vi "gyro_flag.vi"() -> ()   [LabVIEW 2019]
uses:
  <vilib>/Utility/file.llb/Read Delimited Spreadsheet (string).vi
  <vilib>/Analysis/NI_AALBase.lvlib
  <vilib>/Utility/file.llb/Write Delimited Spreadsheet (string).vi
panel:
  out "XY Graph":cluster{timestamp[], "Y":dbl[]}[](graph)
  in  "reset":bool
  out "voltage over time":waveform(dbl)(graph)
  out "charge [V]":dbl
  in  "invert":bool
  out "all rows":string[][](array[string])
  in  "Race time":string
  in  "Other":string
  in  "Enviroment":string(combo)
  in  "Tiredness":string(combo)
  in  "Technique":string(combo)
  in  "Orient":string(combo)
  in  "Ship type":string(combo)
  in  "End Comment":bool
  in  "Type":string(combo)
  in  "?":bool
  in  "Felvesz":bool
  out "csv path":path
  in  "Flag":string(combo)
  out "Timestamp":timestamp
  in  "path to binary file":path=path "C:/Users/Lenovo/Desktop/szakdoga/data"
  # "RESET"
  # "ZOOM"
  # "CURSOR"
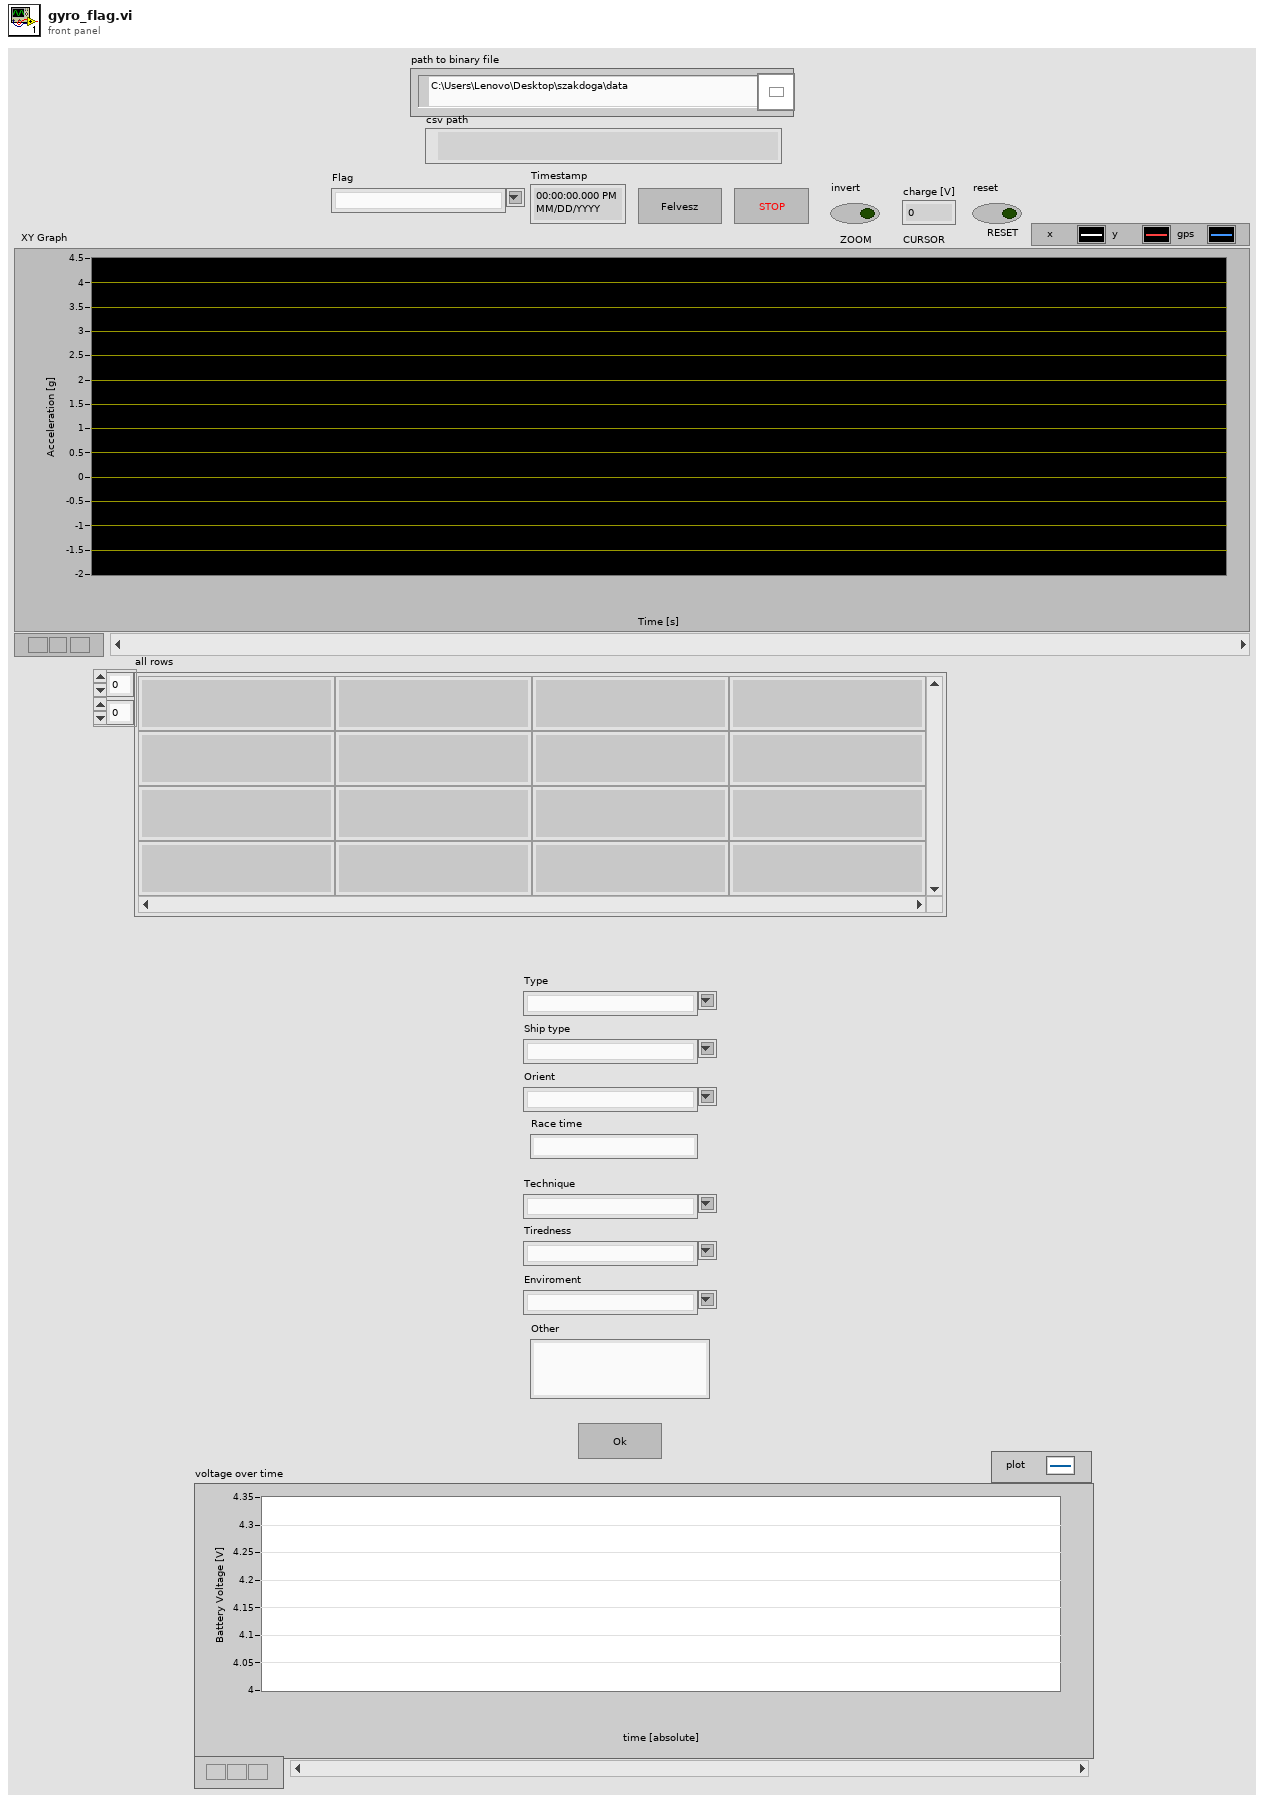
[diagram p1: front panel]
types:
  T1 = enum16{"open", "replace", "create", "open or create", "replace or create", "replace or create with confirmation"}
  T2 = typedef "control_time_informations.ctl" = cluster{"starting time":timestamp, "ending time":timestamp, "dt[s]":dbl, "sampling rate [Hz]":dbl, "length":dbl}
  T3 = typedef "control_all_in_one_package.ctl" = cluster{"memory structure":T4, "actigraph settings":T5, "time informations":T2, "measurement data":T6}
  T4 = typedef "control_memory_structure.ctl" = cluster{"length of metadata [byte]":i32, "length of page [byte]":i32, "length of measurement data on page [byte]":i32, "length of dataset [byte]":i32}
  T5 = typedef "control_measurement_settings.ctl" = cluster{"sampling frequency [Hz]":dbl, "measurement interval [± g]":i32, "high precision?":bool, "number of pages":i32, "rate code":i32, "range code":i32, "id":i32}
  T6 = typedef "control_measurement_data.ctl" = cluster{"number of samples per axis":i32, "timestamp array":dbl[], "offset array":dbl[], "x, y, z axis data":waveform(dbl)[], "normalised magnitude of acceleartion vectors":waveform(dbl), "calibration coefficients":T7, "statistics":T8, "battery voltage":waveform(dbl), "magnitude of acceleartion vectors":waveform(dbl)}
  T7 = typedef "control_calibration_coefficients.ctl" = cluster{"Sx":dbl, "Ox":dbl, "Sy":dbl, "Oy":dbl, "Sz":dbl, "Oz":dbl}
  T8 = typedef "control_statistics.ctl" = cluster{"mean of x axis acceleration":dbl, "standard devation of x axis acceleration":dbl, "mean of y axis acceleration":dbl, "standard devation of y axis acceleration":dbl, "mean of z axis acceleration":dbl, "standard devation of z axis acceleration":dbl, "mean of normalised magnitude of acceleration":dbl, "standard devation of normalised magnitude of acceleration":dbl}
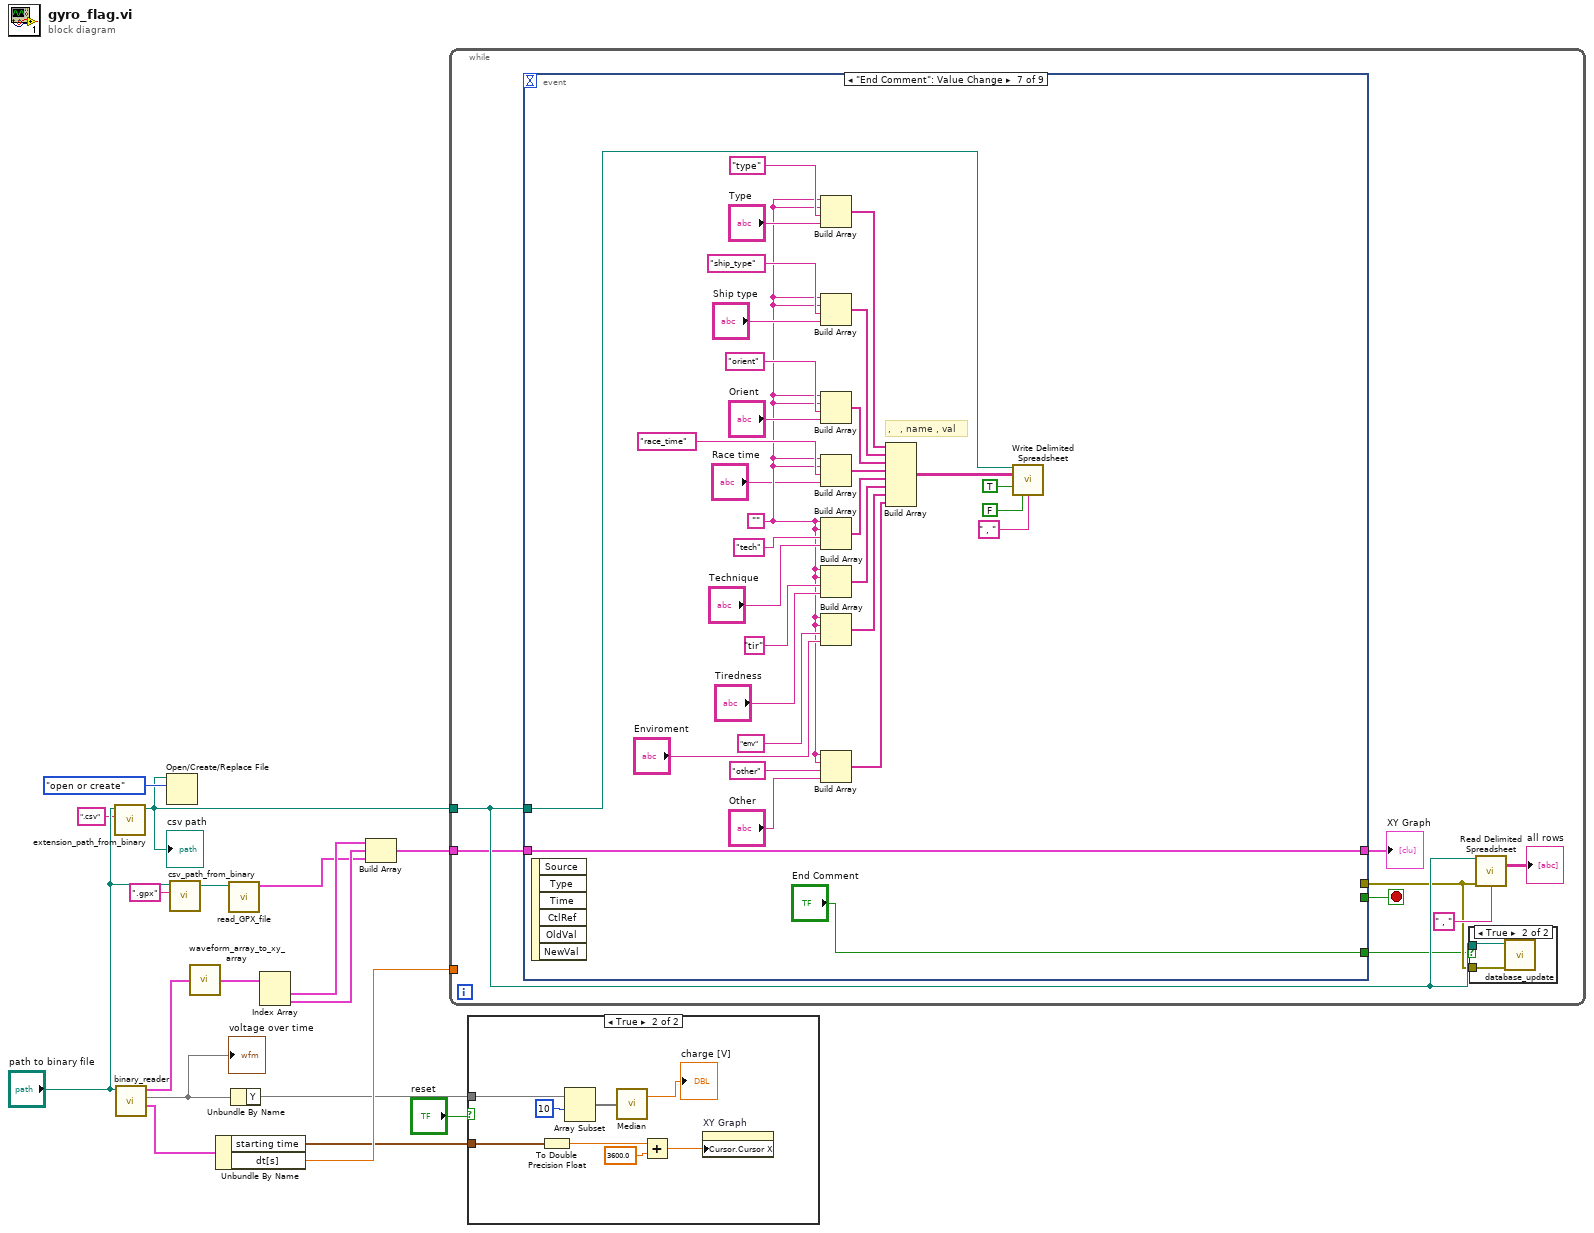
[diagram p0: block diagram]
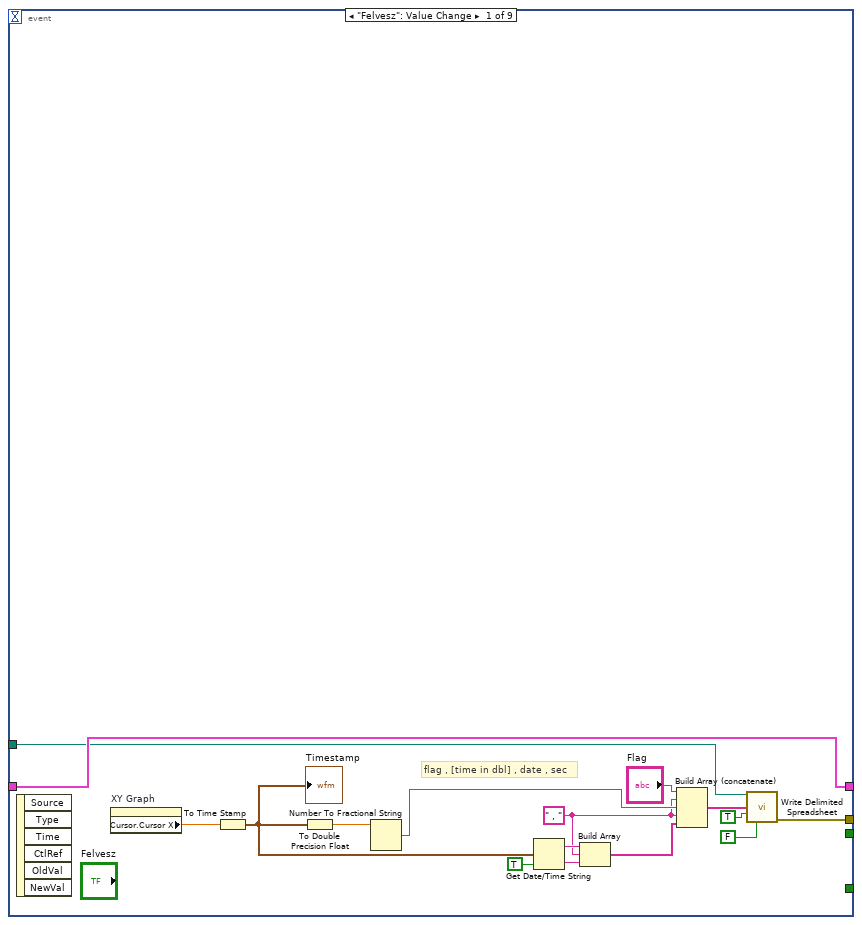
[diagram p4: hidden frame]
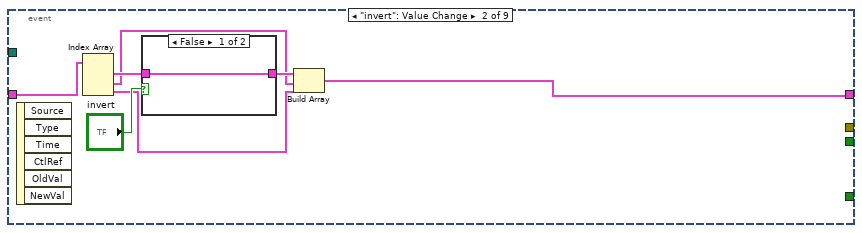
[diagram p5: hidden frame]
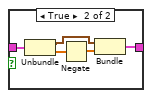
[diagram p6: hidden frame]
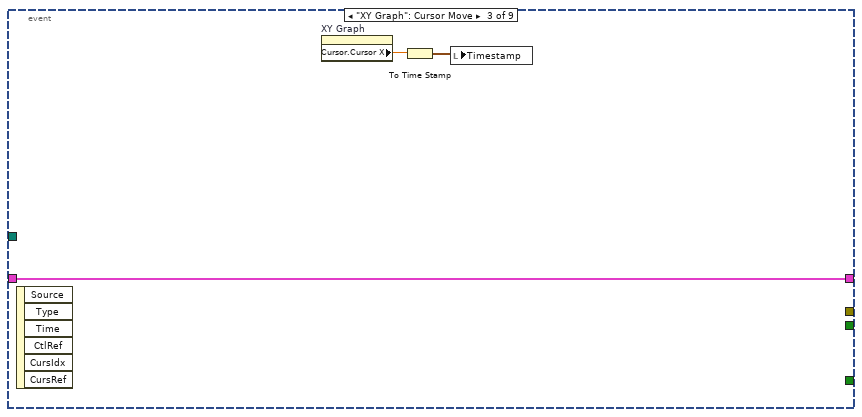
[diagram p7: hidden frame]
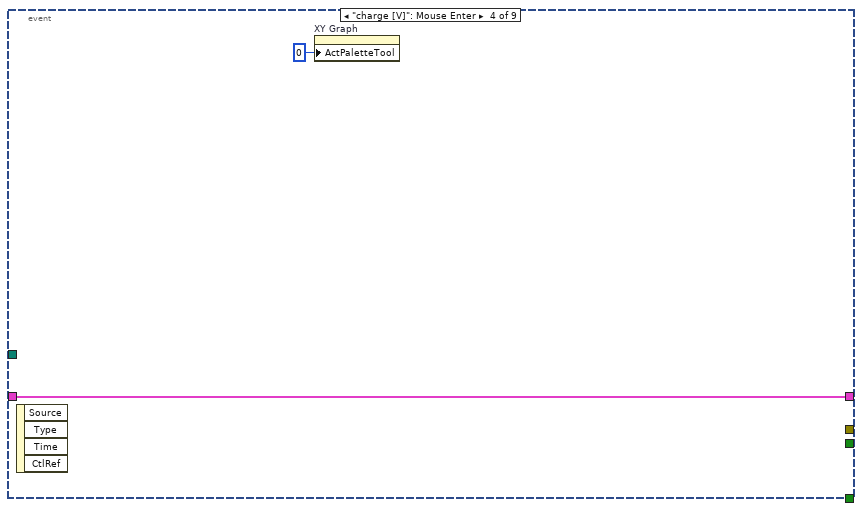
[diagram p8: hidden frame]
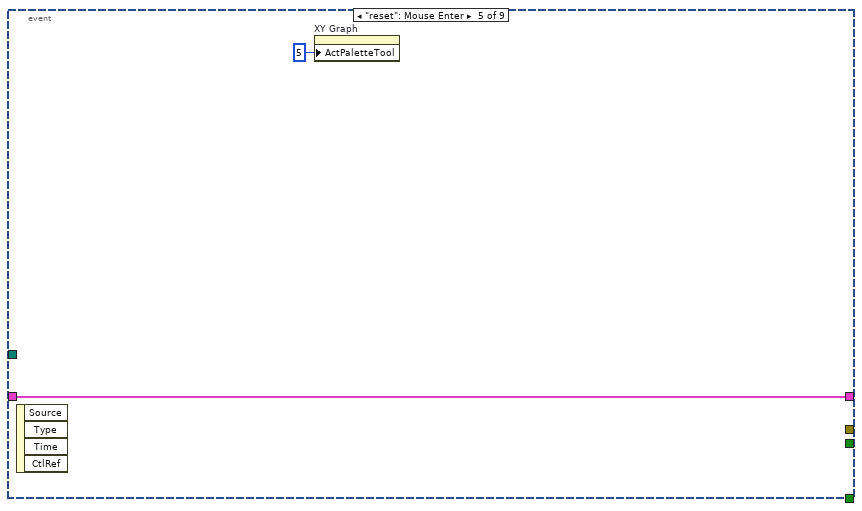
[diagram p9: hidden frame]
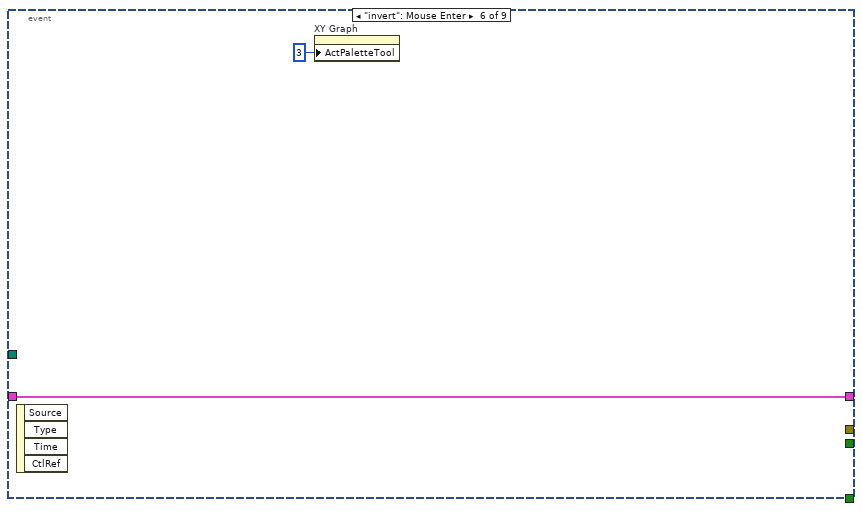
[diagram p10: hidden frame]
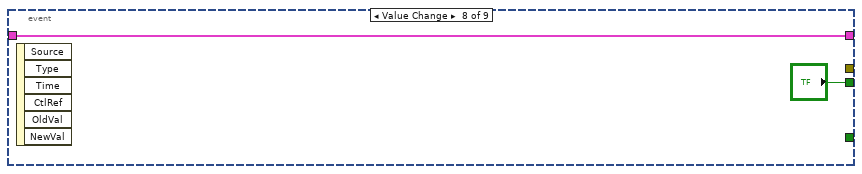
[diagram p11: hidden frame]
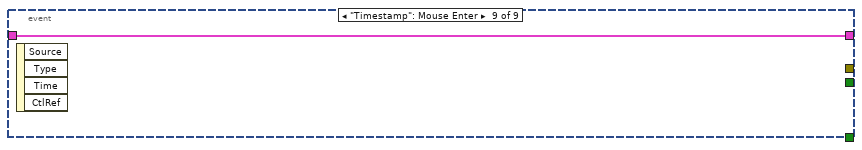
[diagram p12: hidden frame]
diagram:
  n1 = call "extension_path_from_binary.vi"("extension"=".csv", "path to binary file"="path to binary file") -> ("path to csv"=w1:path)  [unwired: 9 in]
  "csv path" <- w1
  n2 = call "binary_reader.vi"("path to binary file"="path to binary file") -> ("time informations"=w12:T2, 2:w11, "all in one package"=w5:T3)  [unwired: 6 in, 1 out]
  "voltage over time" <- w11
  n3 = Open/Create/Replace File(file path (use dialog)=w1, operation (0:open)=T1."open or create") -> ()  [unwired: 4 in, 3 out]
  n4 = call "csv_path_from_binary.vi"("extension"=".gpx", "path to binary file"="path to binary file") -> ("path to spec. ext."=w3:path)  [unwired: 9 in]
  n5 = call "waveform_array_to_xy_array.vi"("waveform array"=w5) -> ("XY array"=w4:cluster{timestamp[], "Y":dbl[]}[])
  n6 = Unbundle By Name(w12) -> ("starting time"=w14:timestamp, "dt[s]"=w16:dbl)
  n7 = call "read_GPX_file.vi"("GPX File Path"=w3) -> ("XY Speed data"=w2:cluster{timestamp[], dbl[]})  [unwired: 3 in, 3 out]
  n8 = Unbundle By Name(w11) -> ("Y"=w10)
  n9 = Index Array(array=w4) -> (element #1=w17:cluster{timestamp[], "Y":dbl[]}, element #2=w15:cluster{timestamp[], "Y":dbl[]})  [unwired: 2 in]
  n10 = Build Array(w17, w15, w2) -> (w13:cluster{timestamp[], "Y":dbl[]}[])
  n11 = while {
    tunnel: w1 -> [w24]
    tunnel: w16 -> [_]
    tunnel: w13 -> [w23]
    stop <- w26 stop-if-true
    n12 = event shown="[6] \"End Comment\": Value Change" {
      selector: _ -> [_ _ _ _ _ _ _ _ _]
      dyn-events: _ -> [_ _ _ _ _ _ _ _ _]
      timeout: _ -> [_ _ _ _ _ _ _ _ _]
      tunnel: [_ _ _ _ _ _ _ "?" _] -> w26
      tunnel: w24 -> [w30 _ _ _ _ _ w96 _ _]
      tunnel: [w29 _ _ _ _ _ _ _ _] -> w22
      tunnel: w23 -> [w31 w51 w58 w61 w63 w65 w68 w99 w101]
      tunnel: [w31 w45 w58 w61 w63 w65 w68 w99 w101] -> w19
      tunnel: [_ _ _ _ _ _ "End Comment" _ _] -> w21
      event "Felvesz": Value Change {
        w38 = " , " ("element")
        # "flag , [time in dbl] , date , sec"
        n13 = event-data() -> ()  [unwired: 1 in, 6 out]
        n14 = property on="XY Graph" class="XYGraph (strict)"() -> ("Cursor.Cursor X"=w33:dbl)  [unwired: 2 in, 2 out]
        n15 = To Time Stamp(1:w33) -> (0:w32:timestamp)
        "Timestamp" <- w32
        n16 = To Double Precision Float(number=w32) -> (double precision float=w43:dbl)
        n17 = Number To Fractional String(number=w43) -> (F-format string=w44:string)  [unwired: 3 in]
        n18 = Get Date/Time String(seconds (now)=w32, want seconds? (F)=TRUE) -> (date string=w40:string, time string=w41:string)  [unwired: 1 in]
        n19 = Build Array(w40, w38, w41) -> (w42:string[])
        n20 = Build Array (concatenate)("Flag", w38, w44, w38, w42) -> (w39:string[])
        n21 = call-poly <vilib>:"Write Delimited Spreadsheet.vi"("file path (dialog if empty)"=w30, "1D data"=w39, "append to file? (new file:F)"=TRUE, "transpose? (no:F)"=FALSE) -> ("error out"=w29:errorcluster)  [unwired: 10 in, 1 out]
      }
      event "invert": Value Change {
        n22 = event-data() -> ()  [unwired: 1 in, 6 out]
        n23 = Index Array(array=w51) -> (element #1=w49:cluster{timestamp[], "Y":dbl[]}, element #2=w47:cluster{timestamp[], "Y":dbl[]}, element #3=w46:cluster{timestamp[], "Y":dbl[]})  [unwired: 3 in]
        n24 = case shown="False" "invert" {
          tunnel: w49 -> [w52 w57]
          tunnel: [w52 w55] -> w48
          frame False {
          }
          frame True {
            n25 = Unbundle(w57) -> (w53:timestamp[], "Y"=w56:dbl[])
            n26 = Negate(x=w56) -> (-x=w54:dbl[])
            n27 = Bundle(w53, w54) -> (w55:cluster{timestamp[], dbl[]})  [unwired: 1 in]
          }
        }
        n28 = Build Array(w48, w47, w46) -> (w45:cluster{timestamp[], "Y":dbl[]}[])
      }
      event "XY Graph": Cursor Move {
        n29 = event-data() -> ()  [unwired: 1 in, 6 out]
        n30 = property on="XY Graph" class="XYGraph (strict)"() -> ("Cursor.Cursor X"=w59:dbl)  [unwired: 2 in, 2 out]
        n31 = To Time Stamp(1:w59) -> (0:w60:timestamp)
        n32 = local write "Timestamp"(w60) -> ()
      }
      event "charge [V]": Mouse Enter {
        n33 = event-data() -> ()  [unwired: 1 in, 4 out]
        n34 = property on="XY Graph" class="XYGraph (strict)"("ActPaletteTool"=0 ("Palette:Active Tool")) -> ()  [unwired: 2 in, 2 out]
      }
      event "reset": Mouse Enter {
        n35 = event-data() -> ()  [unwired: 1 in, 4 out]
        n36 = property on="XY Graph" class="XYGraph (strict)"("ActPaletteTool"=5 ("Palette:Active Tool")) -> ()  [unwired: 2 in, 2 out]
      }
      event "invert": Mouse Enter {
        n37 = event-data() -> ()  [unwired: 1 in, 4 out]
        n38 = property on="XY Graph" class="XYGraph (strict)"("ActPaletteTool"=3 ("Palette:Active Tool")) -> ()  [unwired: 2 in, 2 out]
      }
      event "End Comment": Value Change {
        w72 = ""
        # ",   , name , val"
        n39 = event-data() -> ()  [unwired: 1 in, 6 out]
        n40 = Build Array(w72, w72, "type", "Type") -> (w89:string[])
        n41 = Build Array(w72, w72, "ship_type", "Ship type") -> (w88:string[])
        n42 = Build Array(w72, w72, "orient", "Orient") -> (w78:string[])
        n43 = Build Array(w72, w72, "race_time", "Race time") -> (w77:string[])
        n44 = Build Array(w72, w72, "tech", "Technique") -> (w76:string[])
        n45 = Build Array(w72, w72, "tir", "Tiredness") -> (w75:string[])
        n46 = Build Array(w72, w72, "env", "Enviroment") -> (w74:string[])
        n47 = Build Array(w72, w72, "other", "Other") -> (w69:string[])
        n48 = Build Array(w89, w88, w78, w77, w76, w75, w74, w69) -> (w94:string[][])
        n49 = call-poly <vilib>:"Write Delimited Spreadsheet.vi"("file path (dialog if empty)"=w96, "2D data"=w94, "append to file? (new file:F)"=TRUE, "transpose? (no:F)"=FALSE, "delimiter (\\t)"=" , " ("element")) -> ()  [unwired: 9 in, 2 out]
      }
      event Value Change {
        n50 = event-data() -> ()  [unwired: 1 in, 6 out]
      }
      event "Timestamp": Mouse Enter {
        n51 = event-data() -> ()  [unwired: 1 in, 4 out]
      }
    }
    "XY Graph" <- w19
    n52 = case shown="True" w21 {
      tunnel: w24 -> [_ w28]
      tunnel: w22 -> [_ w27]
      frame False {
      }
      frame True {
        n53 = call "database_update.vi"("error in (no error)"=w27, "path to csv file"=w28) -> ()  [unwired: 10 in]
      }
    }
    n54 = call-poly <vilib>:"Read Delimited Spreadsheet.vi"("file path (dialog if empty)"=w24, "error in (no error)"=w22, "delimiter (\\t)"=" , " ("delimiter (\\t)")) -> ("all rows"=→"all rows":string[][])  [unwired: 7 in, 5 out]
  }
  n55 = case shown="True" "reset" {
    tunnel: w14 -> [_ w107]
    tunnel: w10 -> [_ w106]
    frame False {
    }
    frame True {
      n56 = To Double Precision Float(number=w107) -> (double precision float=w108:dbl)
      n57 = Array Subset(array=w106, index=10) -> (w105:void[])  [unwired: 1 in]
      n58 = call <vilib>:"Median.vi"("X"=w105) -> ("median"=→"charge [V]":dbl)  [unwired: 1 out]
      n59 = Add(x=w108, y=3600.0) -> (x+y=w102:dbl)
      n60 = property on="XY Graph" class="XYGraph (strict)"("Cursor.Cursor X"=w102) -> ()  [unwired: 2 in, 2 out]
    }
  }
